vi "Set Transmission Type.vi"(8 "error in":errorcluster, 10 "Transmission Type":u8(ring)=254 format="%.0x" items=["synchronous (acyclic)"=0, "synchronous (cyclic every sync)"=1, "synchronous (cyclic every 2nd SYNC)"=2, "synchronous (cyclic every 3rd SYNC)"=3, "synchronous (cyclic every 4th SYNC)"=4, "synchronous (cyclic every 240th SYNC)"=240, "reserved"=241, "reserved"=251, "RTR-only (synchronous)"=252, "RTR-only (event-driven)"=253, "event-driven (manufacturer-specific)"=254, "event-driven (device profile and application profile specific)"=255], 11 "TPDO Communication Parameter in":refnum<class "TPDO Communication Parameter.lvclass">) -> (0 "error out":errorcluster, 3 "TPDO Communication Parameter out":refnum<class "TPDO Communication Parameter.lvclass">)   [LabVIEW 2020, in "CANopen.lvlib" / "TPDO Communication Parameter.lvclass"]
uses:
  TPDO Communication Parameter.lvclass
  TPDO Communication Parameter.lvclass/TPDO Communication Parameter.ctl
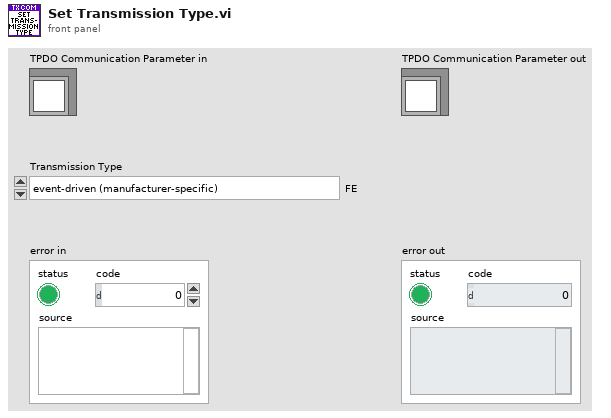
[diagram p1: front panel]
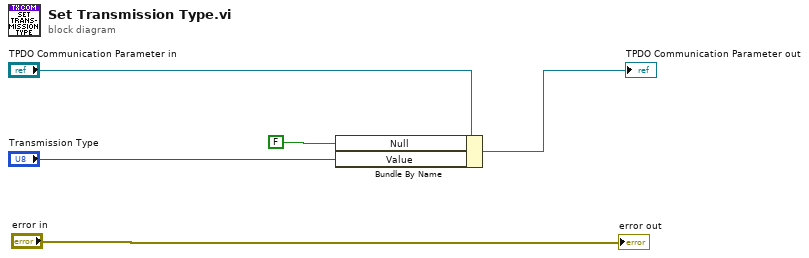
[diagram p0: block diagram]
diagram:
  n1 = Bundle By Name(cluster="TPDO Communication Parameter in", "Null"=FALSE ("Transmission Type.Null"), "Value"="Transmission Type") -> (→"TPDO Communication Parameter out":refnum<class "TPDO Communication Parameter.lvclass">)
  "error out" <- "error in"
